vi "VA CoAP Server.vi"() -> ()   [LabVIEW 2020]
doc: "Creates a named service and listens on the first available port. When a client connects to the service, it sends a response string to the client."
uses:
  <vilib>/addons/JSON API/Variant JSON/Variant JSON.lvlib
  <vilib>/addons/JSON API/JSON Value/JSON Value.lvclass
  data types/MEEB Dock CoAP - Dock - Element - Status.ctl
  data types/MEEB - JSON - Dock.ctl
  data types/VA CoAP - Data Cluster TEST.ctl
  data types/MEEB Dock ID.ctl
  data types/MEEB - JSON - Docks Array.ctl
panel:
  out "JSON":string="{\r  \"Dock\": {\r    \"1\": {\r      \"Command\": \"\",\r      \"Status\": \"\"\r    },\r    \"2\": {\r      \"Command\": \"\",\r      \"Status\": \"\"\r    },\r    \"3\": {\r      \"Command\": \"\",\r      \"Status\": \"\"\r    },\r    \"4\": {\r      \"Command\": \"\",\r      \"Status\": \"\"\r    }\r  }\r}"
  out "error out":errorcluster
  in  "Mem":T1
  in  "Stop":bool
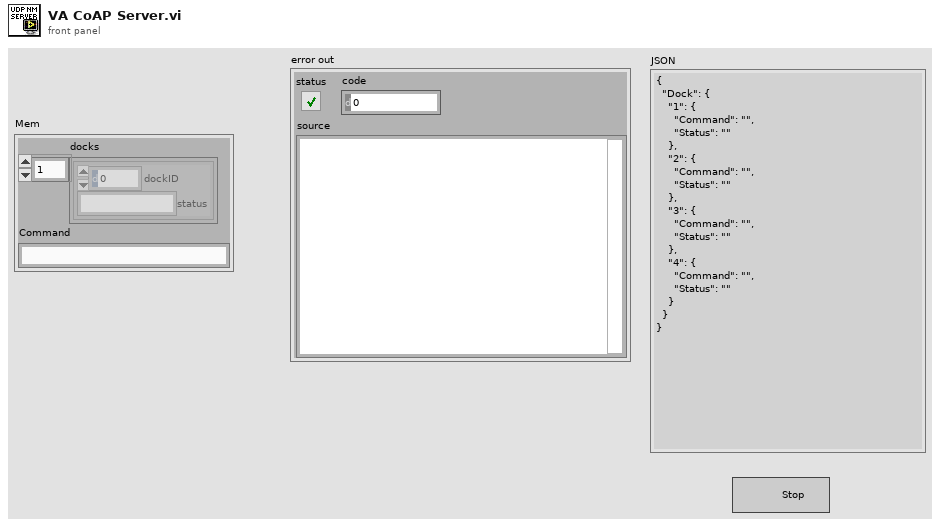
[diagram p1: front panel]
types:
  T1 = typedef "VA CoAP - Data Cluster TEST.ctl" = cluster{"docks":T2, "Command":string}
  T2 = typedef "MEEB - JSON - Docks Array.ctl" = T3[]
  T3 = typedef "MEEB - JSON - Dock.ctl" = cluster{"dockID":T4, "status":T5}
  T4 = typedef "MEEB Dock ID.ctl" = u8
  T5 = typedef "MEEB Dock CoAP - Dock - Element - Status.ctl" = string
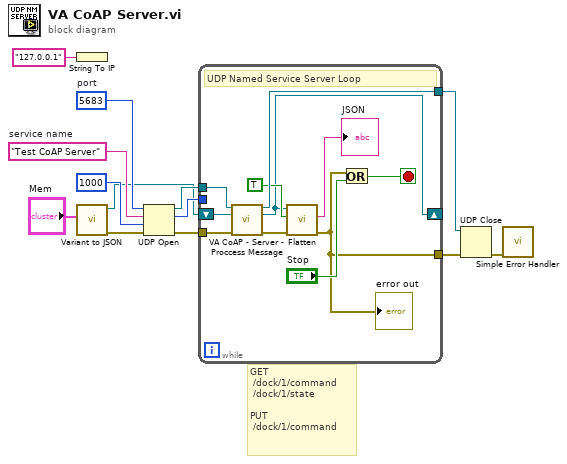
[diagram p0: block diagram]
diagram:
  w7 = u16 5683  # port
  w13 = "Test CoAP Server"  # service name
  # "GET\n /dock/1/command\n /dock/1/state\n\nPUT\n /dock/1/command"
  n1 = String To IP(1:"127.0.0.1") -> ()  [unwired: 1 out]
  n2 = call <vilib>:"Variant to JSON.vi"("Variant"="Mem") -> ("error out"=w3:errorcluster, "JSON Value out"=w1:refnum<class "JSON Value.lvclass">)  [unwired: 9 in]
  n3 = UDP Open(8:w3, 9:1000 ("timeout ms (25000)"), 10:w13, 11:w7) -> (port=w12:refnum<k16>, 0:w11:errorcluster, 2:w9:u16)  [unwired: 1 in]
  n4 = while {
    tunnel: w12 -> [w22]
    tunnel: w11 -> [w20]
    tunnel: w9 -> [_]
    tunnel: [w21] -> w5
    tunnel: [w17] -> w4
    shift-right: [w14] -> _
    shift-left: w1 -> [w19]
    stop <- w24 stop-if-true
    # "UDP Named Service Server Loop"
    n5 = call "VA CoAP - Server - Proccess Message.vi"("Conn IN"=w22, "JSON Value in"=w19, "error in (no error)"=w20) -> ("connection ID out"=w21:refnum<k16>, "JSON Value out"=w14:refnum<class "JSON Value.lvclass">, "error out"=w18:errorcluster)  [unwired: 10 in]
    n6 = call-dynamic "Flatten.vi"("error in (no error)"=w18, "Pretty Print?"=TRUE, "JSON Value in"=w14) -> ("error out"=w17:errorcluster, "<JSON>"=→"JSON":string)  [unwired: 7 in]
    "error out" <- w17
    n7 = Or(x=w17, y="Stop") -> (x .or. y?=w24:bool)
  }
  n8 = UDP Close(connection ID=w5, 8:w4) -> (error out=w8:errorcluster)  [unwired: 1 out]
  n9 = call <vilib>:"Simple Error Handler.vi"("error in (no error)"=w8) -> ()  [unwired: 4 in, 5 out]
